vi "Servo Close N Channels.vi"(8 "Error In":errorcluster, 10 "Servo Channels":u8[](array[numeric]), 11 "LINX Resource":T1) -> (0 "Error Out":errorcluster, 3 "LINX Resource":T1)   [LabVIEW 2011, in "LVH-LINX.lvlib" / "Servo.lvlib"]
doc: "Read the values of the specified digital input channels."
uses:
  Servo.lvlib
  Private/Type Defs/LINX Ref.ctl
  Private/Type Defs/Platform.ctl
  Private/Type Defs/Interface.ctl
  Private/Device/Type Defs/LINX Device Config.ctl
  Private/Device/Type Defs/TCP Config.ctl
  Private/Device/Type Defs/Channels.ctl
  Private/Type Defs/Peripheral.ctl
  Private/Type Defs/Error Type.ctl
  LVH-LINX.lvlib
  Private/Device/Device.lvlib
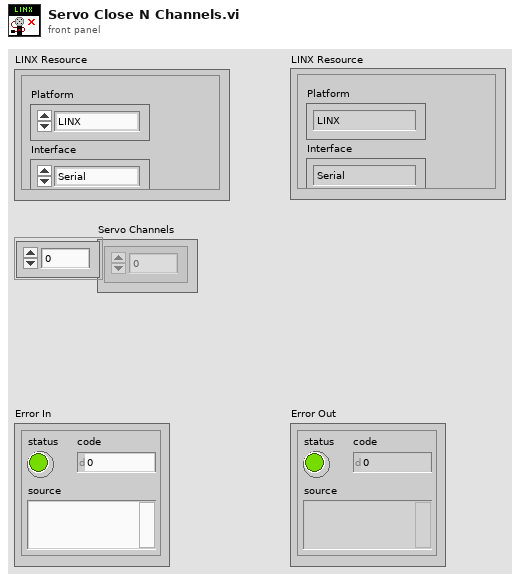
[diagram p1: front panel]
types:
  T1 = typedef "LVH-LINX.lvlib/LINX Ref.ctl" = cluster{"Platform":T2, "Interface":T3, "LINX Device Config":T4}
  T2 = typedef "LVH-LINX.lvlib/Platform.ctl" = enum16{"LINX", "myRIO"}
  T3 = typedef "LVH-LINX.lvlib/Interface.ctl" = enum16{"Serial", "TCP"}
  T4 = typedef "LVH-LINX.lvlib/Device.lvlib/LINX Device Config.ctl" = cluster{"Interface":T3, "COM Port":refnum<visa-resource-name>, "TCP Configuration":T5, "Device Family":u8, "Device ID":u8, "Device Name":string, "TCP Ref":refnum<k5>, "Channels":T6}
  T5 = typedef "LVH-LINX.lvlib/Device.lvlib/TCP Config.ctl" = cluster{"IP Address":string, "Port":u16}
  T6 = typedef "LVH-LINX.lvlib/Channels.ctl" = cluster{"DI":u8[], "DO":u8[], "AI":u8[], "AO":u8[], "PWM":u8[], "QE":u8[], "UART":u8[], "I2C 2":u8[], "SPI":u8[], "CAN":u8[], "Servo":u8[], "AI Ref (V)":dbl, "AO Ref (V)":dbl, "AO Resolution (Bits)":u8}
  T7 = typedef "LVH-LINX.lvlib/Peripheral.ctl" = enum8{"DI", "DO", "AI", "AO", "PWM", "QE", "UART", "I2C", "SPI", "CAN", "Servo"}
  T8 = typedef "LVH-LINX.lvlib/Error Type.ctl" = enum16{"Unknown", "Timeout", "Corrupt Return Packet", "Unable To Connect", "Command Not Supported", "Channel DNE", "Invalid COM Config", "Firmware Version Mismatch", "myRIO Support", "CMD Specific Error"}
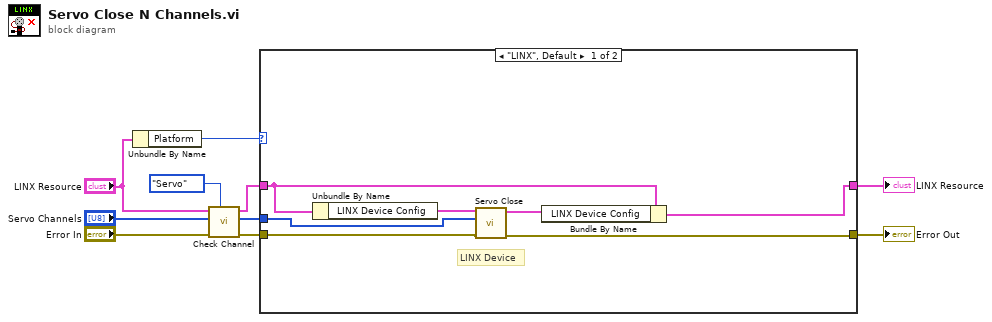
[diagram p0: block diagram]
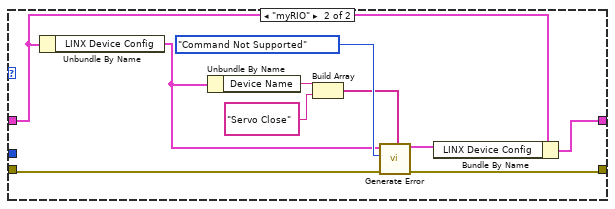
[diagram p2: hidden frame]
diagram:
  n1 = Unbundle By Name("LINX Resource") -> ("Platform"=w10:T2)
  n2 = call "Check Channel.vi"("Peripheral"=Peripheral."Servo", "Error In"="Error In", "Channels"="Servo Channels", "LINX Resource"="LINX Resource") -> ("Error Out"=w7:errorcluster, "Channels"=w6:u8[], "LINX Resource"=w4:T1)  [unwired: 5 in]
  n3 = case shown="\"LINX\", Default" w10 {
    tunnel: w7 -> [w15 w27]
    tunnel: w4 -> [w17 w20]
    tunnel: [w14 w26] -> w9
    tunnel: [w16 w18] -> w8
    tunnel: w6 -> [w13 _]
    frame "LINX", Default {
      # "LINX Device"
      n4 = Unbundle By Name(w17) -> ("LINX Device Config"=w11:T4)
      n5 = call "Servo Close.vi"("Error In"=w15, "Channels"=w13, "LINX Device Config"=w11) -> ("Error Out"=w14:errorcluster, "LINX Device Config"=w12:T4)  [unwired: 7 in]
      n6 = Bundle By Name(cluster=w17, "LINX Device Config"=w12) -> (w16:T1)
    }
    frame "myRIO" {
      n7 = Unbundle By Name(w20) -> ("LINX Device Config"=w21:T4)
      n8 = Unbundle By Name(w21) -> ("Device Name"=w25:string)
      n9 = Build Array(w25, "Servo Close") -> (w22:string[])
      n10 = call "Generate Error.vi"("Error In"=w27, "Arguments"=w22, "Error Type"=Error_Type."Command Not Supported", "LINX Device Config"=w21) -> ("Error Out"=w26:errorcluster, "LINX Device Config"=w19:T4)  [unwired: 6 in]
      n11 = Bundle By Name(cluster=w20, "LINX Device Config"=w19) -> (w18:T1)
    }
  }
  "Error Out" <- w9
  "LINX Resource" <- w8
